vi "Log system error.vi"(8 "error in (no error)":errorcluster, 11 "Channel in":refnum<class "Channel.lvclass">) -> (0 "error out":errorcluster, 3 "Channel out":refnum<class "Channel.lvclass">)   [LabVIEW 2018, in "Channel.lvclass"]
uses:
  Channel.lvclass
  Channel.lvclass/Channel.ctl
  Error log/Error log.lvclass
  Simulated_CCD_Camera/Simulated Camera.lvclass
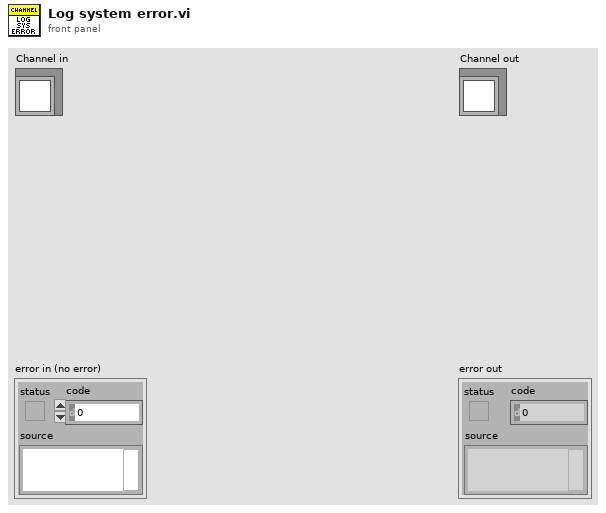
[diagram p1: front panel]
types:
  T1 = cluster{"CYCLES_DONE":u16, "LAST_IMAGE_NAME":string, "DISK_SPACE":u16, "FRAMES_DONE":u16, "CCD_STATUS":string, "CURRENT_TEMPERATURE":i16, "TEMPERATURE_STATUS":string, "FRAME_EXPOSURE_TIME":sgl, "ERROR":bool, "SERIAL_NUMBER":u16, "ACQUIRING":bool, "IMAGE_INDEX":u32, "SEQS_DONE":u16}
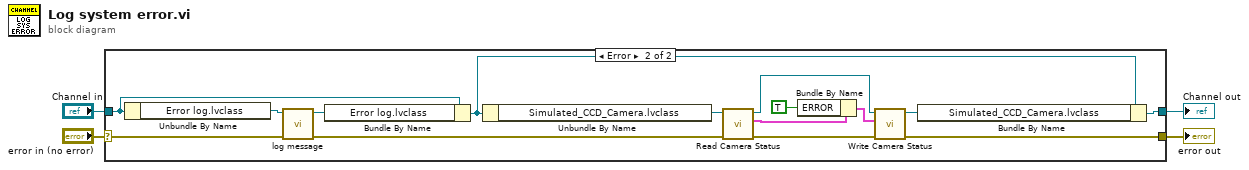
[diagram p0: block diagram]
diagram:
  n1 = case shown="Error" "error in (no error)" {
    selector: "error in (no error)" -> [w6 w20]
    tunnel: [w6 w11] -> w3
    tunnel: [w5 w10] -> w1
    tunnel: "Channel in" -> [w5 w21]
    frame No Error {
    }
    frame Error {
      n2 = Unbundle By Name(w21) -> ("Error log.lvclass"=w18:refnum<class "Error log.lvclass">)
      n3 = call-dynamic "log message.vi"("error in (no error)"=w20, "Error log in"=w18) -> ("error out"=w12:errorcluster, "Error log out"=w19:refnum<class "Error log.lvclass">)  [unwired: 8 in]
      n4 = Bundle By Name(cluster=w21, "Error log.lvclass"=w19) -> (w17:refnum<class "Channel.lvclass">)
      n5 = Unbundle By Name(w17) -> ("Simulated_CCD_Camera.lvclass"=w16:refnum<class "Simulated Camera.lvclass">)
      n6 = call "Read Camera Status.vi"("error in (no error)"=w12, "CCDCamera in"=w16) -> ("error out"=w13:errorcluster, "Camera Status"=w9:T1, "CCDCamera out"=w15:refnum<class "Simulated Camera.lvclass">)  [unwired: 7 in]
      n7 = Bundle By Name(cluster=w9, "ERROR"=TRUE) -> (w8:T1)
      n8 = call "Write Camera Status.vi"("error in (no error)"=w13, "Camera Status"=w8, "CCDCamera in"=w15) -> ("error out"=w11:errorcluster, "CCDCamera out"=w14:refnum<class "Simulated Camera.lvclass">)  [unwired: 7 in]
      n9 = Bundle By Name(cluster=w17, "Simulated_CCD_Camera.lvclass"=w14) -> (w10:refnum<class "Channel.lvclass">)
    }
  }
  "error out" <- w3
  "Channel out" <- w1
